vi "Update Front Panel Instruments.vi"(8 "error in (no error)":errorcluster, 10 "Display References":T1, 11 "Payload Status":T2) -> (0 "error out":errorcluster)   [LabVIEW 2013]
uses:
  Payload Status.ctl
  Intrument References.ctl
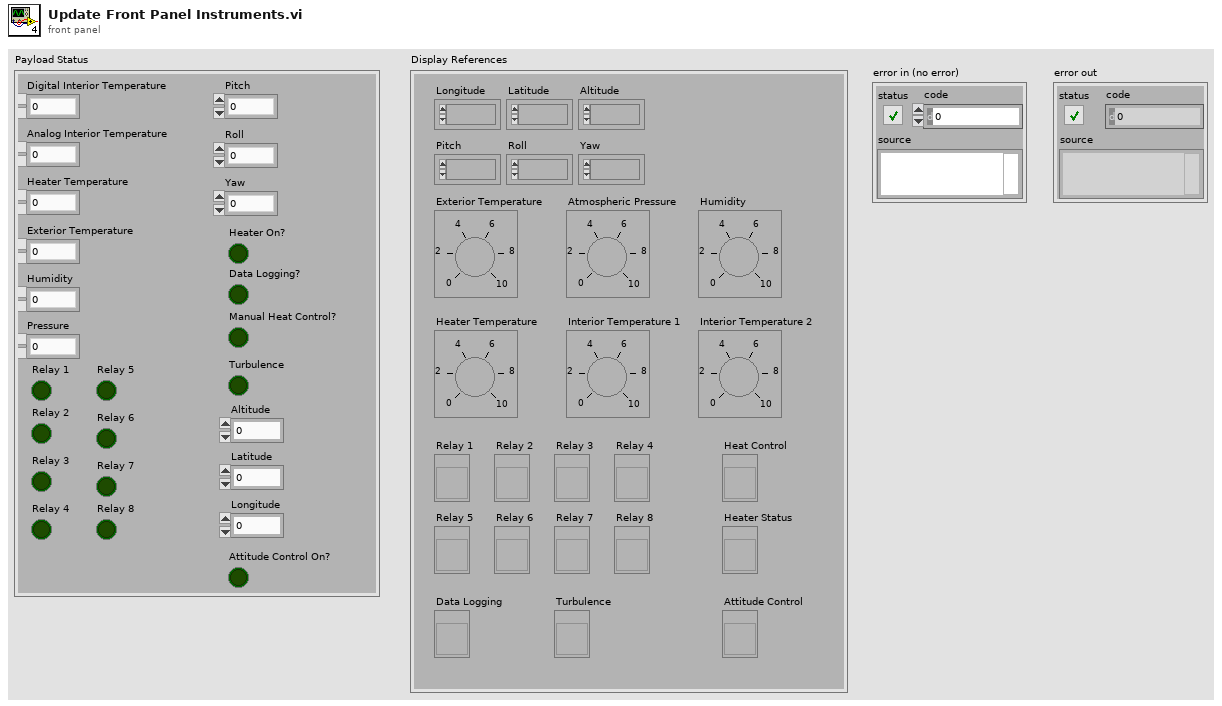
[diagram p1: front panel]
types:
  T1 = typedef "Intrument References.ctl" = cluster{"Latitude":refnum<vi>, "Altitude":refnum<vi>, "Pitch":refnum<vi>, "Roll":refnum<vi>, "Yaw":refnum<vi>, "Humidity":refnum<vi>, "Atmospheric Pressure":refnum<vi>, "Interior Temperature 1":refnum<vi>, "Interior Temperature 2":refnum<vi>, "Exterior Temperature":refnum<vi>, "Heater Temperature":refnum<vi>, "Relay 1":refnum<vi>, "Relay 2":refnum<vi>, "Relay 3":refnum<vi>, "Relay 4":refnum<vi>, "Relay 5":refnum<vi>, "Relay 6":refnum<vi>, "Relay 7":refnum<vi>, "Relay 8":refnum<vi>, "Heat Control":refnum<vi>, "Heater Status":refnum<vi>, "Longitude":refnum<vi>, "Data Logging":refnum<vi>, "Turbulence":refnum<vi>, "Attitude Control":refnum<vi>}
  T2 = typedef "Payload Status.ctl" = cluster{"Digital Interior Temperature":dbl, "Analog Interior Temperature":dbl, "Heater Temperature":dbl, "Exterior Temperature":dbl, "Humidity":dbl, "Pressure":dbl, "Pitch":dbl, "Roll":dbl, "Yaw":dbl, "Heater On?":bool, "Data Logging?":bool, "Manual Heat Control?":bool, "Turbulence":bool, "Relay 1":bool, "Relay 2":bool, "Relay 3":bool, "Relay 4":bool, "Relay 5":bool, "Relay 6":bool, "Relay 7":bool, "Relay 8":bool, "Altitude":dbl, "Latitude":dbl, "Longitude":dbl, "Attitude Control On?":bool}
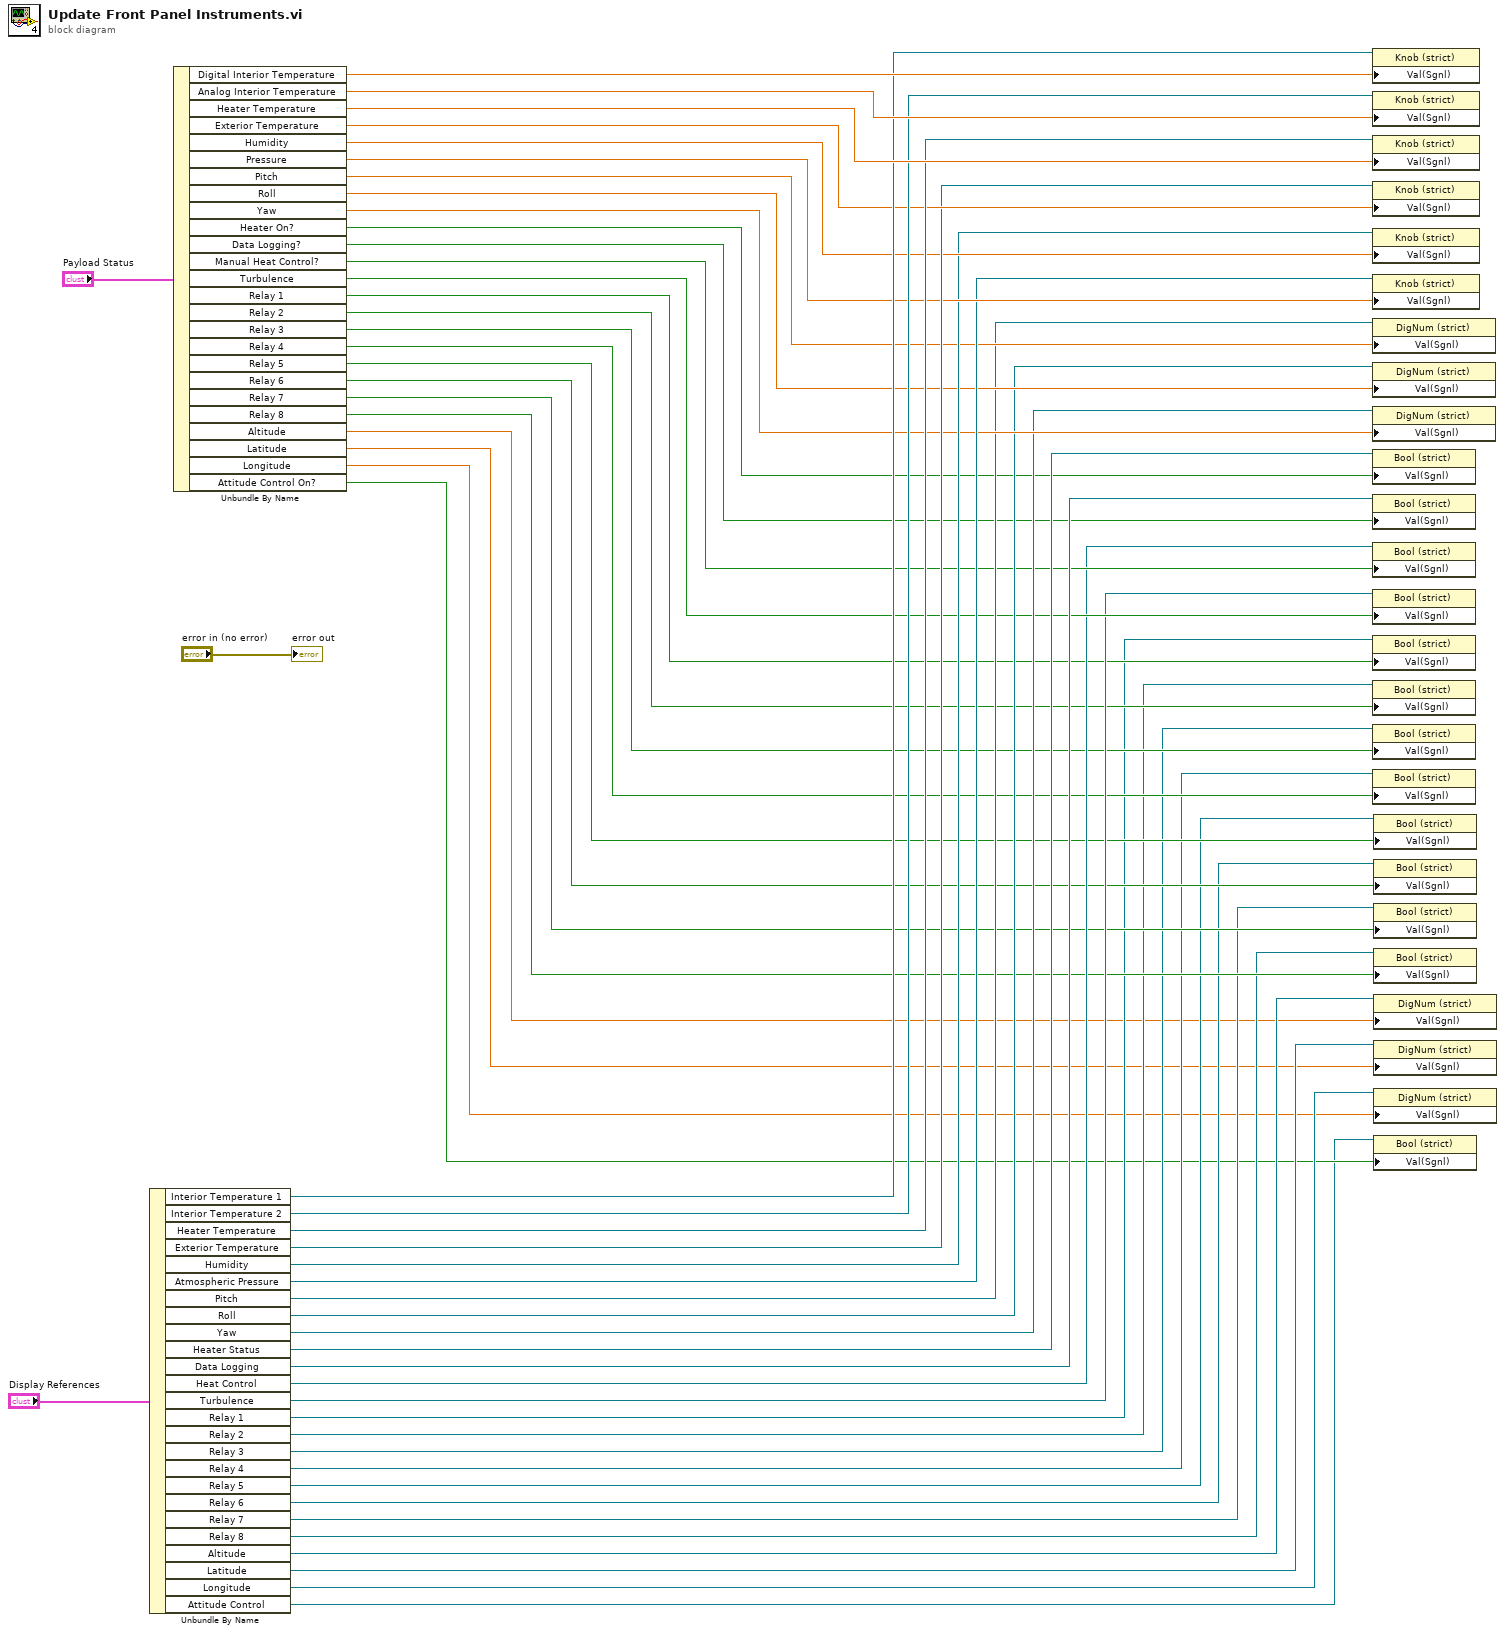
[diagram p0: block diagram]
diagram:
  n1 = Unbundle By Name("Display References") -> ("Interior Temperature 1"=w48:refnum<vi>, "Interior Temperature 2"=w47:refnum<vi>, "Heater Temperature"=w46:refnum<vi>, "Exterior Temperature"=w44:refnum<vi>, "Humidity"=w41:refnum<vi>, "Atmospheric Pressure"=w40:refnum<vi>, "Pitch"=w36:refnum<vi>, "Roll"=w35:refnum<vi>, "Yaw"=w34:refnum<vi>, "Heater Status"=w33:refnum<vi>, "Data Logging"=w32:refnum<vi>, "Heat Control"=w27:refnum<vi>, "Turbulence"=w26:refnum<vi>, "Relay 1"=w17:refnum<vi>, "Relay 2"=w16:refnum<vi>, "Relay 3"=w15:refnum<vi>, "Relay 4"=w14:refnum<vi>, "Relay 5"=w13:refnum<vi>, "Relay 6"=w12:refnum<vi>, "Relay 7"=w11:refnum<vi>, "Relay 8"=w10:refnum<vi>, "Altitude"=w9:refnum<vi>, "Latitude"=w8:refnum<vi>, "Longitude"=w7:refnum<vi>, "Attitude Control"=w1:refnum<vi>)
  n2 = Unbundle By Name("Payload Status") -> ("Digital Interior Temperature"=w51:dbl, "Analog Interior Temperature"=w50:dbl, "Heater Temperature"=w49:dbl, "Exterior Temperature"=w45:dbl, "Humidity"=w43:dbl, "Pressure"=w42:dbl, "Pitch"=w39:dbl, "Roll"=w38:dbl, "Yaw"=w37:dbl, "Heater On?"=w31:bool, "Data Logging?"=w30:bool, "Manual Heat Control?"=w29:bool, "Turbulence"=w28:bool, "Relay 1"=w25:bool, "Relay 2"=w24:bool, "Relay 3"=w23:bool, "Relay 4"=w22:bool, "Relay 5"=w21:bool, "Relay 6"=w20:bool, "Relay 7"=w19:bool, "Relay 8"=w18:bool, "Altitude"=w6:dbl, "Latitude"=w5:dbl, "Longitude"=w4:dbl, "Attitude Control On?"=w2:bool)
  n3 = property class="Knob (strict)"(reference=w48, "Val(Sgnl)"=w51) -> ()  [unwired: 1 in, 2 out]
  n4 = property class="Knob (strict)"(reference=w47, "Val(Sgnl)"=w50) -> ()  [unwired: 1 in, 2 out]
  n5 = property class="Knob (strict)"(reference=w46, "Val(Sgnl)"=w49) -> ()  [unwired: 1 in, 2 out]
  n6 = property class="Knob (strict)"(reference=w44, "Val(Sgnl)"=w45) -> ()  [unwired: 1 in, 2 out]
  n7 = property class="Knob (strict)"(reference=w41, "Val(Sgnl)"=w43) -> ()  [unwired: 1 in, 2 out]
  n8 = property class="Knob (strict)"(reference=w40, "Val(Sgnl)"=w42) -> ()  [unwired: 1 in, 2 out]
  n9 = property class="DigNum (strict)"(reference=w36, "Val(Sgnl)"=w39) -> ()  [unwired: 1 in, 2 out]
  n10 = property class="DigNum (strict)"(reference=w35, "Val(Sgnl)"=w38) -> ()  [unwired: 1 in, 2 out]
  n11 = property class="DigNum (strict)"(reference=w34, "Val(Sgnl)"=w37) -> ()  [unwired: 1 in, 2 out]
  n12 = property class="Bool (strict)"(reference=w33, "Val(Sgnl)"=w31) -> ()  [unwired: 1 in, 2 out]
  n13 = property class="Bool (strict)"(reference=w32, "Val(Sgnl)"=w30) -> ()  [unwired: 1 in, 2 out]
  n14 = property class="Bool (strict)"(reference=w27, "Val(Sgnl)"=w29) -> ()  [unwired: 1 in, 2 out]
  n15 = property class="Bool (strict)"(reference=w26, "Val(Sgnl)"=w28) -> ()  [unwired: 1 in, 2 out]
  n16 = property class="Bool (strict)"(reference=w17, "Val(Sgnl)"=w25) -> ()  [unwired: 1 in, 2 out]
  n17 = property class="Bool (strict)"(reference=w16, "Val(Sgnl)"=w24) -> ()  [unwired: 1 in, 2 out]
  n18 = property class="Bool (strict)"(reference=w15, "Val(Sgnl)"=w23) -> ()  [unwired: 1 in, 2 out]
  n19 = property class="Bool (strict)"(reference=w14, "Val(Sgnl)"=w22) -> ()  [unwired: 1 in, 2 out]
  n20 = property class="Bool (strict)"(reference=w13, "Val(Sgnl)"=w21) -> ()  [unwired: 1 in, 2 out]
  n21 = property class="Bool (strict)"(reference=w12, "Val(Sgnl)"=w20) -> ()  [unwired: 1 in, 2 out]
  n22 = property class="Bool (strict)"(reference=w11, "Val(Sgnl)"=w19) -> ()  [unwired: 1 in, 2 out]
  n23 = property class="Bool (strict)"(reference=w10, "Val(Sgnl)"=w18) -> ()  [unwired: 1 in, 2 out]
  n24 = property class="DigNum (strict)"(reference=w9, "Val(Sgnl)"=w6) -> ()  [unwired: 1 in, 2 out]
  n25 = property class="DigNum (strict)"(reference=w8, "Val(Sgnl)"=w5) -> ()  [unwired: 1 in, 2 out]
  n26 = property class="DigNum (strict)"(reference=w7, "Val(Sgnl)"=w4) -> ()  [unwired: 1 in, 2 out]
  n27 = property class="Bool (strict)"(reference=w1, "Val(Sgnl)"=w2) -> ()  [unwired: 1 in, 2 out]
  "error out" <- "error in (no error)"
